vi "run.vi"(8 "error in (no error)":errorcluster, 11 "TCPServer in":refnum<class "TCPServer.lvclass">) -> (0 "error out":errorcluster, 3 "TCPServer out":refnum<class "TCPServer.lvclass">)   [LabVIEW 2016, in "TCPServer.lvclass"]
uses:
  TCPServer.lvclass
  C:/Users/aanania/Documents/ts_monochromator_windows/ts_labview_tcp/TCPCommunicator/TCPCommunicator.lvclass
  TCPCommunicator/TCPCommunicator.lvclass/TCPCommunicator.ctl
  TCPComEvents/TCPComEvents.lvclass/TCPComEvents.ctl
  TCPComEvents/TCPComEvents.lvclass
  TCPCommunicator/TCPCommunicator.lvclass
panel:
  out "stop":bool
  out "remote address":string
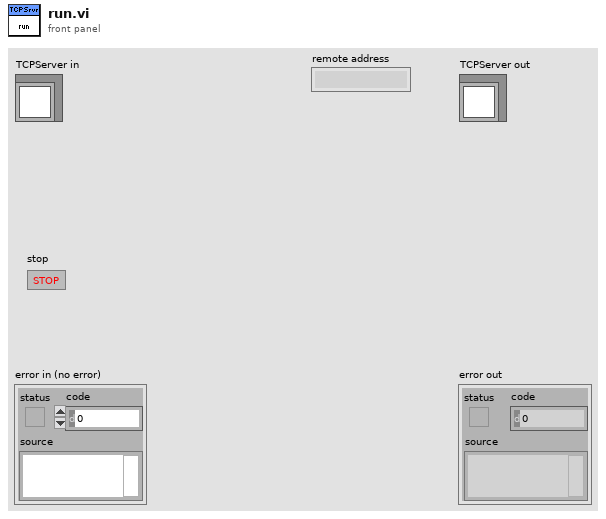
[diagram p1: front panel]
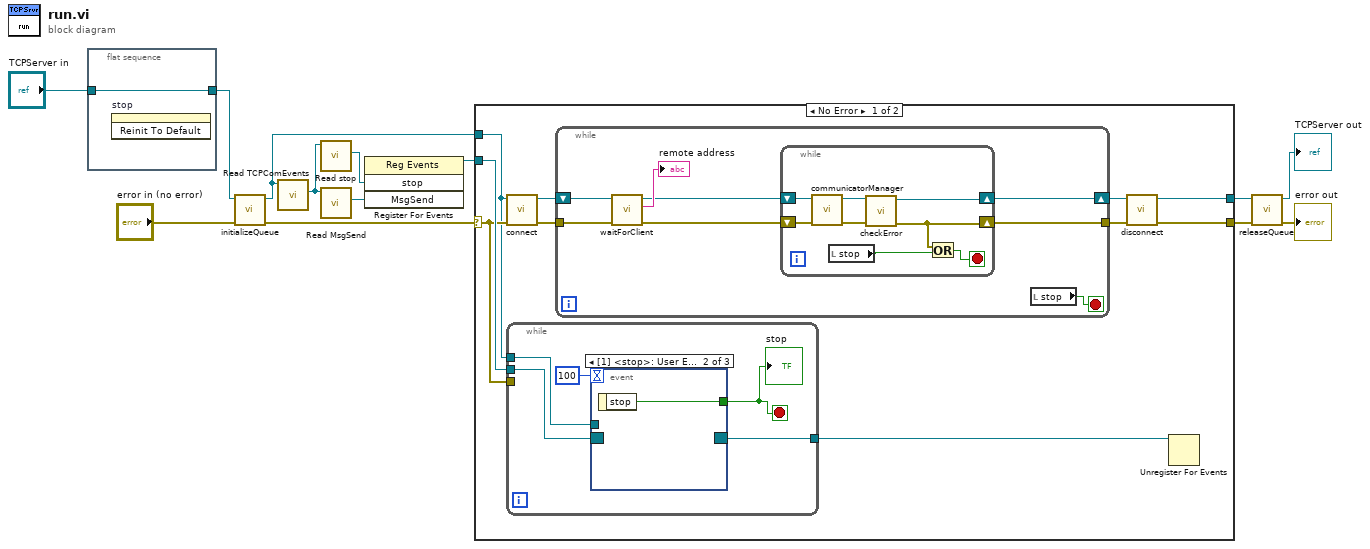
[diagram p0: block diagram]
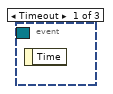
[diagram p2: hidden frame]
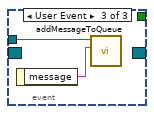
[diagram p3: hidden frame]
diagram:
  n1 = flat-sequence {
    tunnel: [w14] -> w10
    tunnel: "TCPServer in" -> [w14]
    frame #0 {
      n2 = invoke on="stop" class="Bool (strict)" method="Reinit To Default"() -> ()  [unwired: 3 in, 3 out]
    }
  }
  n3 = call-dynamic "initializeQueue.vi"("error in (no error)"="error in (no error)", "TCPCommunicator in"=w10) -> ("error out"=w7:errorcluster, "TCPCommunicator out"=w9:refnum<class "TCPServer.lvclass">)  [unwired: 8 in]
  n4 = call "Read TCPComEvents.vi"("TCPCommunicator in"=w9) -> ("TCPComEvents.lvclass"=w2:refnum<class "TCPComEvents.lvclass">)  [unwired: 8 in, 2 out]
  n5 = call "Read stop.vi"("TCPComEvents in"=w2) -> ("stop"=w13:refnum<user-event>)  [unwired: 8 in, 2 out]
  n6 = call "Read MsgSend.vi"("TCPComEvents in"=w2) -> ("MsgSend"=w1:refnum<user-event>)  [unwired: 8 in, 2 out]
  n7 = register-events(w13, w1) -> (reference out=w12:refnum<event-registration>)  [unwired: 2 in, 1 out]
  n8 = case shown="No Error" w7 {
    selector: w7 -> [w22 w50]
    tunnel: [w18 w50] -> w5
    tunnel: [w16 w49] -> w6
    tunnel: w9 -> [w15 w49]
    tunnel: w12 -> [w24 _]
    frame No Error {
      n9 = call-dynamic "connect.vi"("error in (no error)"=w22, "TCPServer in"=w15) -> ("error out"=w21:errorcluster, "TCPServer out"=w23:refnum<class "TCPServer.lvclass">)  [unwired: 8 in]
      n10 = while {
        tunnel: w22 -> [_]
        tunnel: w24 -> [w28]
        tunnel: [w27] -> w20
        tunnel: w15 -> [w26]
        stop <- w25 stop-if-true
        n11 = event shown="[1] <stop>: User Event" {
          selector: w28 -> [_ _ _]
          dyn-events: [_ _ _] -> w27
          timeout: 100 -> [_ _ _]
          tunnel: [_ w30 _] -> w25
          tunnel: w26 -> [_ _ w32]
          event Timeout {
            n12 = event-data() -> ()  [unwired: 1 in, 1 out]
          }
          event User Event {
            n13 = event-data() -> ("stop"=w30:bool)  [unwired: 1 in]
          }
          event User Event {
            n14 = event-data() -> ("message"=w31:string)  [unwired: 1 in]
            n15 = call-dynamic "addMessageToQueue.vi"("message"=w31, "TCPCommunicator in"=w32) -> ()  [unwired: 7 in, 3 out]
          }
        }
        "stop" <- w25
      }
      n16 = while {
        shift-right: [w34] -> w17
        shift-left: w23 -> [w40]
        tunnel: w21 -> [w39]
        tunnel: [w35] -> w19
        stop <- w33 stop-if-true
        n17 = call "waitForClient.vi"("error in (no error)"=w39, "TCPServer in"=w40) -> ("error out"=w37:errorcluster, "remote address"=→"remote address":string, "TCPServer out"=w36:refnum<class "TCPServer.lvclass">)  [unwired: 6 in, 1 out]
        n18 = while {
          shift-right: [w43] -> w35
          shift-left: w37 -> [w48]
          shift-right: [w44] -> w34
          shift-left: w36 -> [w47]
          stop <- w42 stop-if-true
          n19 = call "communicatorManager.vi"("error in (no error)"=w48, "TCPServer in"=w47) -> ("error out"=w46:errorcluster, "TCPServer out"=w45:refnum<class "TCPServer.lvclass">)  [unwired: 8 in]
          n20 = local read "stop"() -> (w41:bool)
          n21 = call "checkError.vi"("error in (no error)"=w46, "TCPServer in"=w45) -> ("error out"=w43:errorcluster, "TCPServer out"=w44:refnum<class "TCPServer.lvclass">)  [unwired: 7 in, 1 out]
          n22 = Or(x=w43, y=w41) -> (x .or. y?=w42:bool)
        }
        n23 = local read "stop"() -> (w33:bool)
      }
      n24 = call-dynamic "disconnect.vi"("error in (no error)"=w19, "TCPServer in"=w17) -> ("error out"=w18:errorcluster, "TCPServer out"=w16:refnum<class "TCPServer.lvclass">)  [unwired: 8 in]
      n25 = Unregister For Events(event registration refnum=w20) -> ()  [unwired: 1 in, 1 out]
    }
    frame Error {
    }
  }
  n26 = call-dynamic "releaseQueue.vi"("error in (no error)"=w5, "TCPCommunicator in"=w6) -> ("error out"=→"error out":errorcluster, "TCPCommunicator out"=→"TCPServer out":refnum<class "TCPServer.lvclass">)  [unwired: 8 in]
